vi "Configure DC Volts.vi"(0 "VISA resource name":refnum<visa-resource-name>, 1 "Enable Auto Range (T:Enable)":bool=TRUE, 3 "Auto-zero (1: On)":u16(ring)=1 format="%.0g" items=["Off", "On", "Once"], 4 "Manual Range (0 V)":dbl format="%#_6p", 5 "error in (no error)":errorcluster, 6 "Power Line Cycles (1.00)":dbl=1.0 min=0.0005 max=100.0 format="%.2f", 7 "Sampling Interval (0.05)":dbl=0.05 min=0.0002 max=3600.0 step=0.0001 format="%.4f", 9 "Input Impedance (0: Hi-Z)":u16(ring) format="%.0g" items=["Hi-Z", "10M Ohm"], 12 "Digits (5: 5 1/2)":u16(ring)=5 format="%.0g" items=["3 1/2 Digits"=3, "4 1/2 Digits"=4, "5 1/2 Digits"=5]) -> (14 "VISA resource name out":refnum<visa-resource-name>, 19 "error out":errorcluster)   [LabVIEW 2017, in "ADCMT7451_ADC.lvlib"]
doc: "Configures the measurement type, resolution, and range on the instrument."
uses:
  ADCMT7451_ADC.lvlib
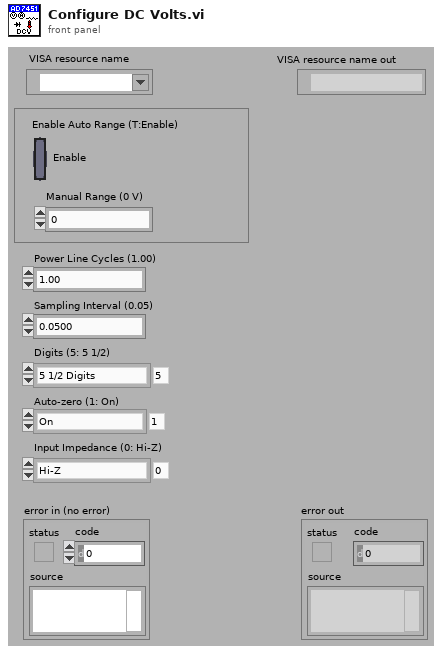
[diagram p1: front panel]
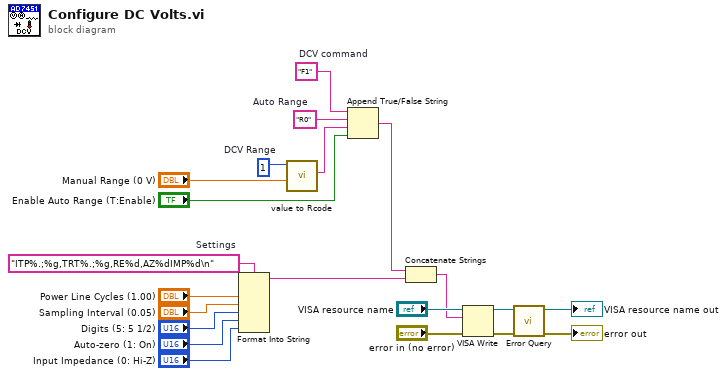
[diagram p0: block diagram]
diagram:
  w8 = "ITP%.;%g,TRT%.;%g,RE%d,AZ%dIMP%d\n"  # Settings
  w1 = 1  # DCV Range
  w11 = "F1"  # DCV command
  w14 = "R0"  # Auto Range
  n1 = Format Into String(format string=w8, "Power Line Cycles (1.00)", "Sampling Interval (0.05)", "Digits (5: 5 1/2)", "Auto-zero (1: On)", "Input Impedance (0: Hi-Z)") -> (resulting string=w2:string)  [unwired: 2 in, 1 out]
  n2 = call "value to Rcode.vi"("Manual Range (0)"="Manual Range (0 V)", "Function (1: DC Volts)"=w1) -> ("Range Set Code"=w9:string)  [unwired: 9 in]
  n3 = Append True/False String(1:"Enable Auto Range (T:Enable)", 2:w9, 3:w14, 4:w11) -> (0:w13:string)
  n4 = Concatenate Strings(w13, w2) -> (w12:string)
  n5 = VISA Write(VISA resource name="VISA resource name", write buffer=w12, error in (no error)="error in (no error)") -> (VISA resource name out=w17:refnum<visa-resource-name>, error out=w16:errorcluster)  [unwired: 1 out]
  n6 = call "Error Query.vi"("error in (no error)"=w16, "VISA resource name"=w17) -> ("error out"=→"error out":errorcluster, "VISA resource name out"=→"VISA resource name out":refnum<visa-resource-name>)  [unwired: 6 in, 2 out]
